vi "Thread@KeySectionUnLock__Parameter.vi"(1 "ParamterIn":string) -> (0 "ParamterOut":string)   [LabVIEW 2020]
panel:
  in  "Locker":string(combo)
  in  "Confirm":bool
  # "Thread@Lock $UnLocker"
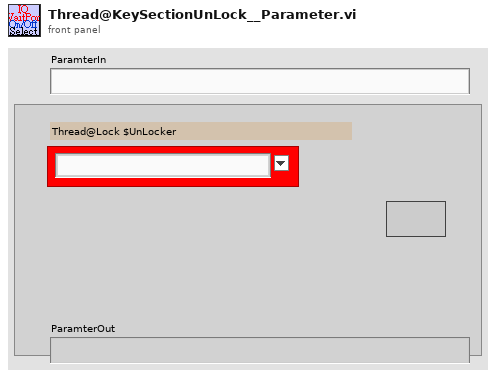
[diagram p1: front panel]
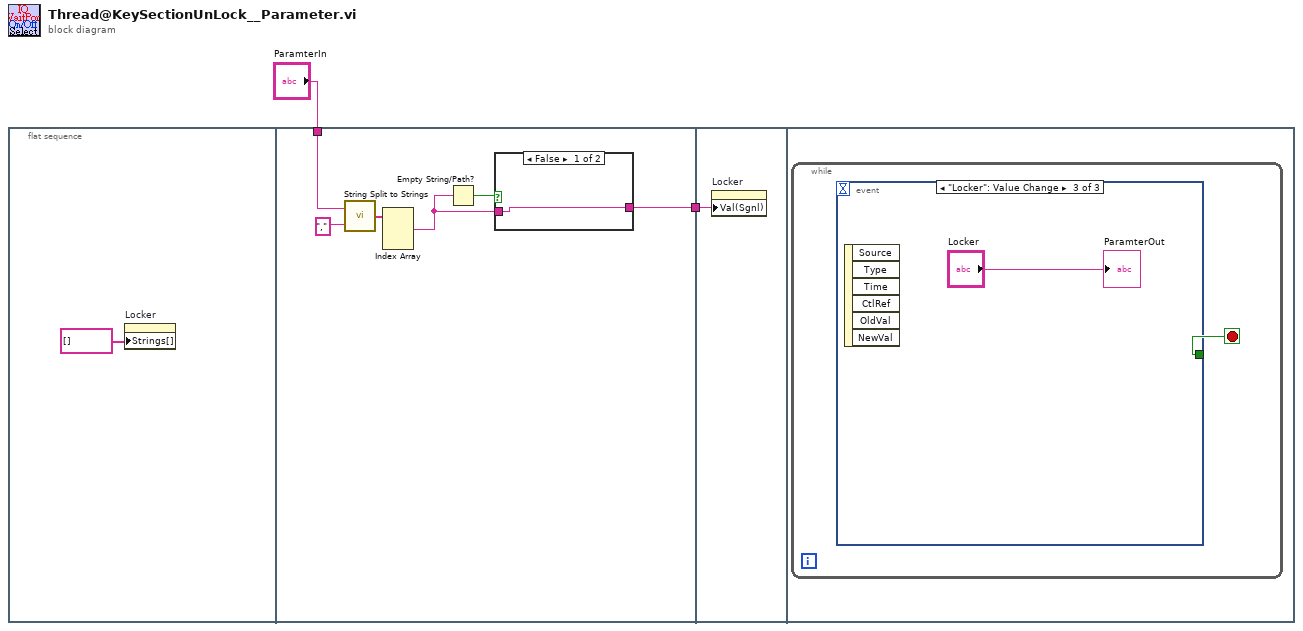
[diagram p0: block diagram]
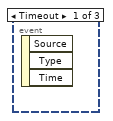
[diagram p3: hidden frame]
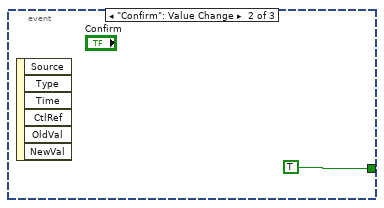
[diagram p4: hidden frame]
diagram:
  n1 = flat-sequence {
    tunnel: "ParamterIn" -> [w7]
    tunnel: [w4] -> w1
    tunnel: w1 -> [w11]
    frame #0 {
      n2 = property on="Locker" class="CmbBox"("Strings[]"=string[] [] ("Strings []")) -> ()  [unwired: 2 in, 2 out]
    }
    frame #1 {
      n3 = call "String Split to Strings.vi"("search string/char (-)"=",", "String"=w7) -> ("Array"=w9:string[])
      n4 = Index Array(array=w9) -> (element #1=w5:string)  [unwired: 3 in, 2 out]
      n5 = Empty String/Path?(string/path=w5) -> (empty?=w6:bool)
      n6 = case shown="False" w6 {
        tunnel: w5 -> [w10 _]
        tunnel: [w10 _] -> w4
        frame False {
        }
        frame True {
        }
      }
    }
    frame #2 {
      n7 = property on="Locker" class="CmbBox"("Val(Sgnl)"=w11) -> ()  [unwired: 2 in, 2 out]
    }
    frame #3 {
      n8 = while {
        stop <- w12 stop-if-true
        n9 = event shown="[2] \"Locker\": Value Change" {
          selector: _ -> [_ _ _]
          dyn-events: _ -> [_ _ _]
          timeout: _ -> [_ _ _]
          tunnel: [_ TRUE _] -> w12
          event Timeout {
            n10 = event-data() -> ()  [unwired: 1 in, 3 out]
          }
          event "Confirm": Value Change {
            n11 = event-data() -> ()  [unwired: 1 in, 6 out]
          }
          event "Locker": Value Change {
            n12 = event-data() -> ()  [unwired: 1 in, 6 out]
            "ParamterOut" <- "Locker"
          }
        }
      }
    }
  }
